vi "Tag Test.vi"() -> ()   [LabVIEW 2024]
uses:
  <vilib>/Skyline/Tag/Shared/typedefs/DataType.ctl
  <vilib>/Skyline/Utilities/Build Resource Name.vi
  <vilib>/Skyline/Configuration/Configuration HTTP_class/Open Configuration HTTP Auto.vi
  <vilib>/Skyline/Tag/Wrapper/Wrapper_class/Write Tag (DBL).vi
  <vilib>/Skyline/Tag/Wrapper/Wrapper_class/Close Tag (Single).vi
  <vilib>/Skyline/Tag/Wrapper/Wrapper HTTP_class/NI Skyline Tag HTTP.lvclass
  <vilib>/Skyline/Tag/Wrapper/Wrapper_class/NI Skyline Tag.lvclass
  <vilib>/Skyline/Tag/Shared/NI Skyline Tag.lvlib
  <vilib>/Skyline/Configuration/Configuration HTTP_class/NI Skyline Configuration HTTP.lvclass
panel:
  out "error out":errorcluster
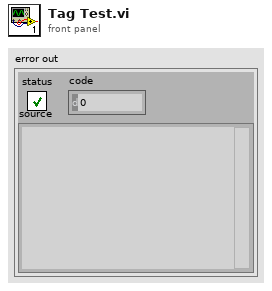
[diagram p1: front panel]
types:
  T1 = typedef "NI Skyline Tag.lvlib/DataType.ctl" = enum32{"Double", "I32", "String", "Boolean", "U64", "Timestamp"}
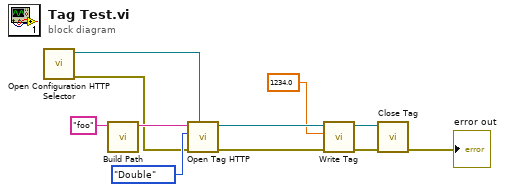
[diagram p0: block diagram]
diagram:
  n1 = call-poly <vilib>:"Open Configuration HTTP Selector.vi"() -> ("error out"=w1:errorcluster, "configuration"=w2:refnum<class "NI Skyline Configuration HTTP.lvclass">)  [unwired: 10 in]
  n2 = call <vilib>:"Build Path.vi"("tag name"="foo") -> ("path"=w11:string)  [unwired: 10 in]
  n3 = call <vilib>:"Open Tag HTTP.vi"("configuration"=w2, "error in (no error)"=w1, "Data Type"=DataType."Double", "path"=w11) -> ("error out"=w7:errorcluster, "tag"=w10:refnum<class "NI Skyline Tag.lvclass">)  [unwired: 6 in]
  n4 = call-poly <vilib>:"Write Tag.vi"("error in (no error)"=w7, "value"=1234.0, "tag in"=w10) -> ("error out"=w8:errorcluster, "tag out"=w9:refnum<class "NI Skyline Tag.lvclass">)  [unwired: 7 in]
  n5 = call-poly <vilib>:"Close Tag.vi"("error in (no error)"=w8, "tag"=w9) -> ("error out"=→"error out":errorcluster)  [unwired: 9 in]
